vi "CoincidenceHist.vi"(1 "delayed channel":u8, 2 "length (µs)":dbl format="%.2f", 3 "range":cluster{"x0":dbl, "x1":dbl} {"x1" format="%.2f"; "x0" format="%.2f"}, 4 "input rawdata":T1) -> (0 "coincidence histogram":T2={"origin (ns)"=0.0, "offset (ns)"=100.0, "histogram"=[]} {"offset (ns)" format="%.2f"; "origin (ns)" format="%.2f"})   [LabVIEW 2009]
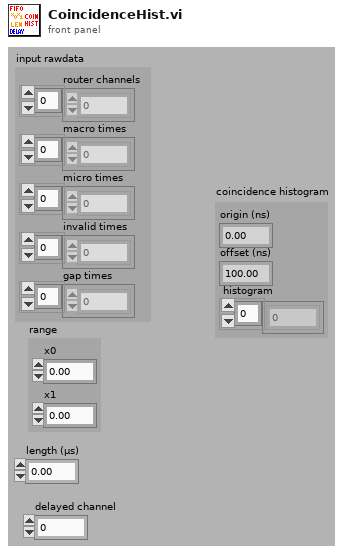
[diagram p1: front panel]
types:
  T1 = cluster{"router channels":u8[], "macro times":u32[], "micro times":u16[], "invalid times":u32[], "gap times":u32[]}
  T2 = cluster{"origin (ns)":dbl, "offset (ns)":dbl, "histogram":u32[]}
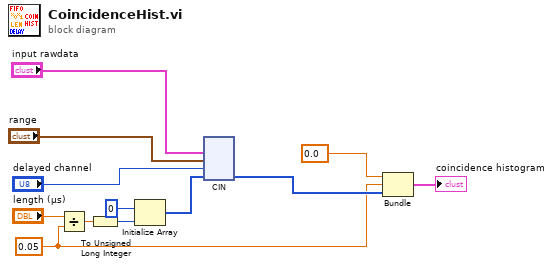
[diagram p0: block diagram]
diagram:
  w4 = 0.05 ("y")
  n1 = Divide(x="length (µs)", y=w4) -> (x/y=w9:dbl)
  n2 = To Unsigned Long Integer(number=w9) -> (unsigned 32bit integer=w8:u32)
  n3 = Initialize Array(u32 0 ("element"), w8) -> (w6:u32[])
  n4 = cin("input rawdata", "range", "delayed channel", w6) -> (w5:u32[])  [unwired: 3 in]
  n5 = Bundle(0.0, "y"=w4, w5) -> (→"coincidence histogram":cluster{dbl, "y":dbl, u32[]})  [unwired: 1 in]
